vi "Get Wheel Parameter by Name as String.vi"(8 "error in (no error)":errorcluster, 10 "parameter name":string, 11 "wheel in":refnum<class "NI_Robotics_Wheel.lvclass">) -> (0 "error out":errorcluster, 1 "found?":bool, 2 "parameter value":string, 3 "wheel out":refnum<class "NI_Robotics_Wheel.lvclass">)   [LabVIEW 2017, in "NI_Robotics_Wheel.lvclass"]
uses:
  <vilib>/robotics/Steering/Wheel/NI_Robotics_Wheel.lvclass
  <vilib>/robotics/Steering/Wheel/NI_Robotics_Wheel.lvclass/NI_Robotics_Wheel.ctl
  <vilib>/robotics/Actuation/Motor Communication/NI_Robotics_Motor Communication.lvclass/NI_Robotics_Motor Communication.ctl
  <vilib>/robotics/Actuation/Motor Communication/NI_Robotics_Motor Communication.lvclass
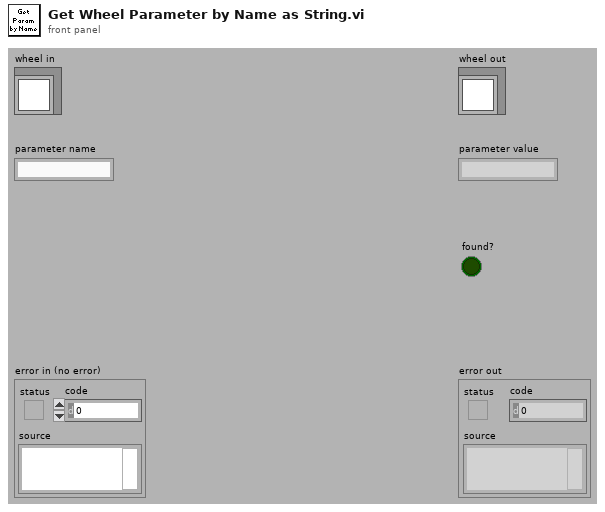
[diagram p1: front panel]
types:
  T1 = typedef "NI_Robotics_Wheel.lvclass/Rotation Direction.ctl" = u16
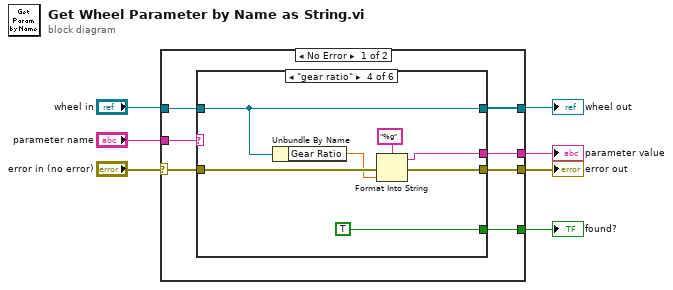
[diagram p0: block diagram]
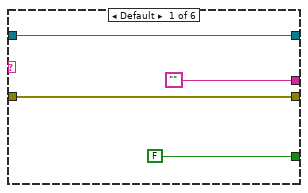
[diagram p2: hidden frame]
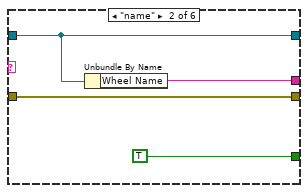
[diagram p3: hidden frame]
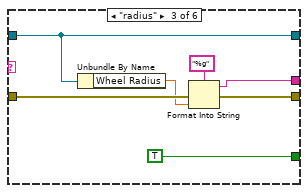
[diagram p4: hidden frame]
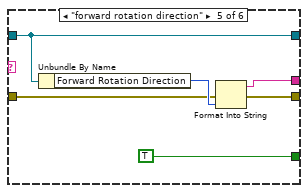
[diagram p5: hidden frame]
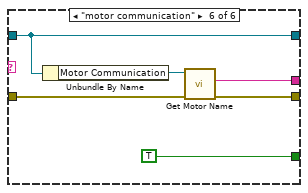
[diagram p6: hidden frame]
diagram:
  n1 = case shown="No Error" "error in (no error)" {
    selector: "error in (no error)" -> [w9 w50]
    tunnel: [w8 w50] -> w3
    tunnel: [w12 w49] -> w6
    tunnel: "wheel in" -> [w13 w49]
    tunnel: "parameter name" -> [w14 _]
    tunnel: [w11 _] -> w1
    tunnel: [w10 _] -> w5
    frame No Error {
      n2 = case shown="\"gear ratio\"" w14 {
        tunnel: w13 -> [w18 w22 w29 w36 w42 w48]
        tunnel: [w18 w22 w29 w36 w42 w48] -> w12
        tunnel: ["" w21 w24 w31 w37 w45] -> w11
        tunnel: [FALSE TRUE TRUE TRUE TRUE TRUE] -> w10
        tunnel: [w15 w19 w26 w33 w38 w44] -> w8
        tunnel: w9 -> [w15 w19 w27 w34 w39 w43]
        frame Default {
        }
        frame "name" {
          n3 = Unbundle By Name(w22) -> ("Wheel Name"=w21:string)
        }
        frame "radius" {
          n4 = Unbundle By Name(w29) -> ("Wheel Radius"=w25:dbl)
          n5 = Format Into String(format string="%g", error in=w27, w25) -> (resulting string=w24:string, error out=w26:errorcluster)  [unwired: 1 in]
        }
        frame "gear ratio" {
          n6 = Unbundle By Name(w36) -> ("Gear Ratio"=w32:dbl)
          n7 = Format Into String(format string="%g", error in=w34, w32) -> (resulting string=w31:string, error out=w33:errorcluster)  [unwired: 1 in]
        }
        frame "forward rotation direction" {
          n8 = Unbundle By Name(w42) -> ("Forward Rotation Direction"=w40:T1)
          n9 = Format Into String(error in=w39, w40) -> (resulting string=w37:string, error out=w38:errorcluster)  [unwired: 2 in]
        }
        frame "motor communication" {
          n10 = Unbundle By Name(w48) -> ("Motor Communication"=w46:refnum<class "NI_Robotics_Motor Communication.lvclass">)
          n11 = call <vilib>:"Get Motor Name.vi"("error in (no error)"=w43, "motor communication in"=w46) -> ("error out"=w44:errorcluster, "motor name"=w45:string)  [unwired: 7 in, 1 out]
        }
      }
    }
    frame Error {
    }
  }
  "error out" <- w3
  "wheel out" <- w6
  "found?" <- w5
  "parameter value" <- w1
